vi "AlliGator Plugin Target to Submenu.vi"(9 "Function Target Type":T1, 11 "Function Target":string) -> (3 "Menu Tag":string)   [LabVIEW 2021, in "AlliGator Python Plugins.lvlib"]
doc: "Convert Plugin Target to Menu Tag for insertion of the menu item.\n\nFor plugins associated with objects such as Source Image or Decay Graph, the insertion takes place at the bottom of contextual menu and thus an empty string is provided.\n\nFor plugins associated with data not exposed to the user (such as the Gate Series), the plugin menui is added to the main menu, and thus the tag of the submenu in which it will be inserted needs to be provided."
uses:
  AlliGator Python Plugins.lvlib
  AlliGator Python Plugin Target Type.ctl
panel:
  # "see the AlliGator License on the block diagram (Ctrl+E or Window:Show Block Diagram)"
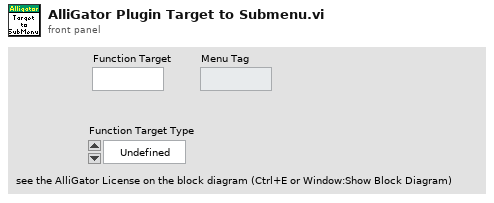
[diagram p1: front panel]
types:
  T1 = typedef "AlliGator Python Plugins.lvlib/AlliGator Python Plugin Target Type.ctl" = enum16{"Undefined", "Window Menu", "Object Menu"}
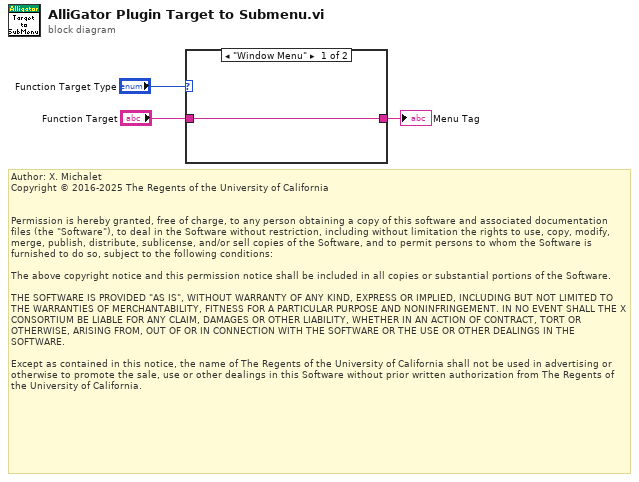
[diagram p0: block diagram]
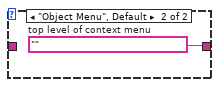
[diagram p2: hidden frame]
diagram:
  # "Author: X. Michalet\nCopyright © 2016-2025 The Regents of the University of California\n \n\nPermission is hereby granted, free of charge, to any person obtaining a copy of this software and associated documentation files (the \"Software\"), to deal in the Software without restriction, including without limitation the rights to use, copy, modify, merge, publish, distribute, sublicense, and/or sell copies of the Software, and to permit persons to whom the Software is furnished to do so, subject to the following conditions:\n\nThe above copyright notice and this permission notice shall be included in all copies or substantial portions of the Software.\n\nTHE SOFTWARE IS PROVIDED \"AS IS\", WITHOUT WARRANTY OF ANY KIND, EXPRESS OR IMPLIED, INCLUDING BUT NOT LIMITED TO THE WARRANTIES OF MERCHANTABILITY, FITNESS FOR A PARTICULAR PURPOSE AND NONINFRINGEMENT. IN NO EVENT SHALL THE X CONSORTIUM BE LIABLE FOR ANY CLAIM, DAMAGES OR OTHER LIABILITY, WHETHER IN AN ACTION OF CONTRACT, TORT OR OTHERWISE, ARISING FROM, OUT OF OR IN CONNECTION WITH THE SOFTWARE OR THE USE OR OTHER DEALINGS IN THE SOFTWARE.\n\nExcept as contained in this notice, the name of The Regents of the University of California shall not be used in advertising or otherwise to promote the sale, use or other dealings in this Software without prior written authorization from The Regents of the University of California."
  n1 = case shown="\"Window Menu\"" "Function Target Type" {
    tunnel: "Function Target" -> [w4 _]
    tunnel: [w4 w5] -> w1
    frame "Window Menu" {
    }
    frame "Object Menu", Default {
      w5 = ""  # top level of context menu
    }
  }
  "Menu Tag" <- w1
